vi "Generate SysDef Path.vi"() -> (0 "System Definition path":path)   [LabVIEW 2018, in "FPGA Addon Scalar Channels System Tests.lvclass"]
uses:
  FPGA Addon Scalar Channels System Tests.lvclass
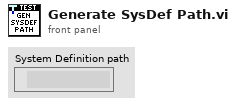
[diagram p1: front panel]
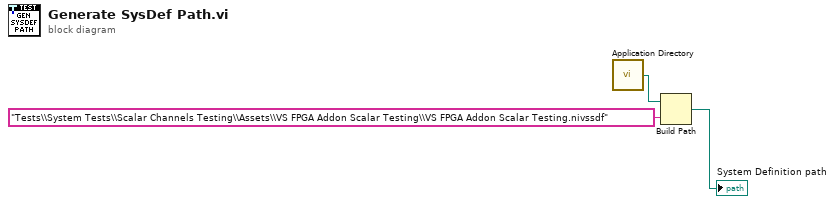
[diagram p0: block diagram]
diagram:
  n1 = call <vilib>:"Application Directory.vi"() -> ("Application Directory"=w1:path)
  n2 = Build Path(base path=w1, name or relative path="Tests\\System Tests\\Scalar Channels Testing\\Assets\\VS FPGA Addon Scalar Testing\\VS FPGA Addon Scalar Testing.nivssdf") -> (appended path=→"System Definition path":path)
